vi "Refresh is Frame Not in ECU.vi"(7 "ECU Name":string, 8 "Type (Input)":T3, 9 "Frame":T1, 10 "Frames":T1[](array[typedef]), 11 "ECUs":T4[](array[typedef])) -> (3 "True?":bool)   [LabVIEW 2020, in "Communication Bus Template System Explorer.lvlib" / "Implementation.lvlib"]
uses:
  Implementation.lvlib
  Types/ECU.ctl
  <vilib>/NI VeriStand/Custom Device API/Custom Device Channel Type.ctl
  Types/Frame.ctl
  Types/Signal.ctl
  <vilib>/NI VeriStand/Custom Device API/Custom Device API.lvlib
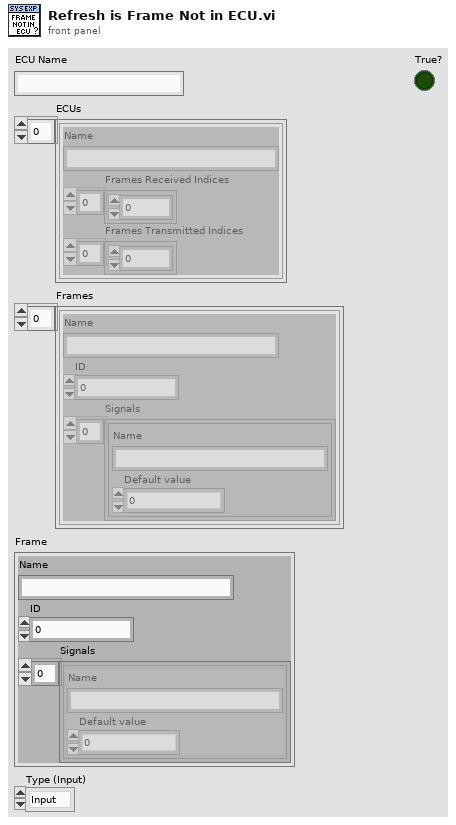
[diagram p1: front panel]
types:
  T1 = typedef "Communication Bus Template System Explorer.lvlib/Implementation.lvlib/Frame.ctl" = cluster{"Name":string, "ID":u32, "Signals":T2[]}
  T2 = typedef "Communication Bus Template System Explorer.lvlib/Implementation.lvlib/Signal.ctl" = cluster{"Name":string, "Default value":dbl}
  T3 = typedef "Custom Device API.lvlib/Custom Device Channel Type.ctl" = enum16{"Input", "Output"}
  T4 = typedef "Communication Bus Template System Explorer.lvlib/Implementation.lvlib/ECU.ctl" = cluster{"Name":string, "Frames Received Indices":u32[], "Frames Transmitted Indices":u32[]}
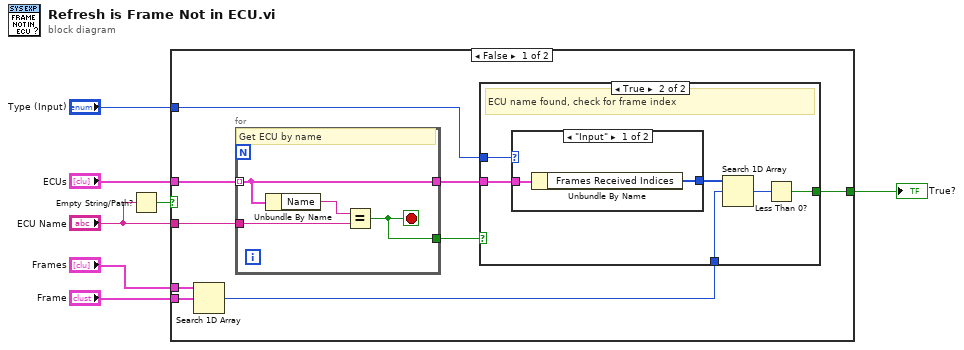
[diagram p0: block diagram]
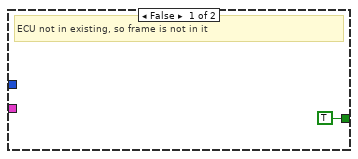
[diagram p2: hidden frame]
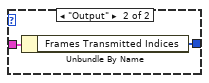
[diagram p3: hidden frame]
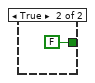
[diagram p4: hidden frame]
diagram:
  n1 = Empty String/Path?(string/path="ECU Name") -> (empty?=w2:bool)
  n2 = case shown="False" w2 {
    tunnel: "Frames" -> [w16 _]
    tunnel: "Frame" -> [w15 _]
    tunnel: "ECUs" -> [w14 _]
    tunnel: "ECU Name" -> [w13 _]
    tunnel: "Type (Input)" -> [w12 _]
    tunnel: [w8 FALSE] -> w3
    frame False {
      n3 = Search 1D Array(1D array=w16, element=w15) -> (index of element=w10:i32)  [unwired: 1 in]
      n4 = for {
        tunnel: w14 -> [w29] mode=indexing
        tunnel: w13 -> [w30]
        tunnel: [w29] -> w11
        tunnel: [w28] -> w9
        stop <- w28 stop-if-true
        # "Get ECU by name"
        n5 = Unbundle By Name(w29) -> ("Name"=w31:string)
        n6 = Equal?(x=w31, y=w30) -> (x = y?=w28:bool)
      }
      n7 = case shown="True" w9 {
        tunnel: w12 -> [_ w21]
        tunnel: w11 -> [_ w20]
        tunnel: w10 -> [_ w19]
        tunnel: [TRUE w18] -> w8
        frame False {
          # "ECU not in existing, so frame is not in it"
        }
        frame True {
          # "ECU name found, check for frame index"
          n8 = case shown="\"Input\"" w21 {
            tunnel: w20 -> [w25 w27]
            tunnel: [w24 w26] -> w22
            frame "Input" {
              n9 = Unbundle By Name(w25) -> ("Frames Received Indices"=w24:u32[])
            }
            frame "Output" {
              n10 = Unbundle By Name(w27) -> ("Frames Transmitted Indices"=w26:u32[])
            }
          }
          n11 = Search 1D Array(1D array=w22, element=w19) -> (index of element=w23:i32)  [unwired: 1 in]
          n12 = Less Than 0?(x=w23) -> (x < 0?=w18:bool)
        }
      }
    }
    frame True {
    }
  }
  "True?" <- w3
